vi "GetWindowParent.vi"(8 "No Error":errorcluster, 11 "Window [SDL_Window *]":i64) -> (0 "error out":errorcluster, 3 "Parent Window [SDL_Window *]":i64)   [LabVIEW 2024, in "SDL3.lvlib" / "Video.lvlib"]
doc: "<B>Summary</B>\nGet parent of a window."
uses:
  Video.lvlib
  Lib/SDL3-32.dll
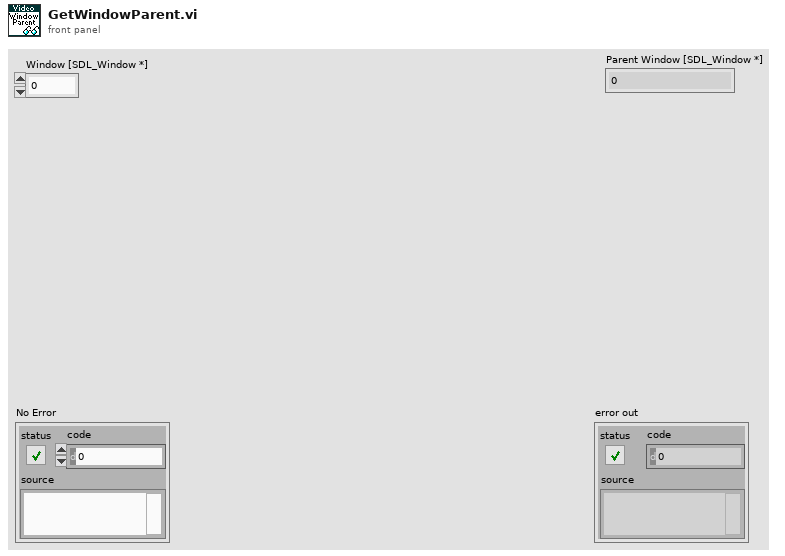
[diagram p1: front panel]
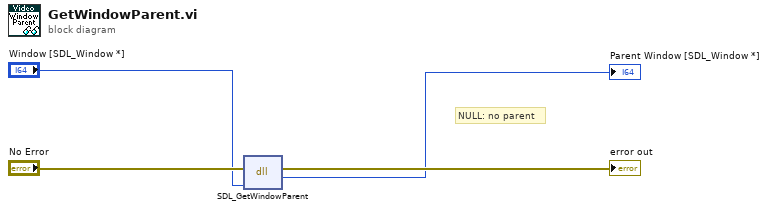
[diagram p0: block diagram]
diagram:
  # "NULL: no parent"
  n1 = dll-call lib="C:/Users/Thomas/Documents/Projects/LV-SDL3/Lib/SDL3-*.*" fn="SDL_GetWindowParent"(error in="No Error", "window"="Window [SDL_Window *]") -> (error out=→"error out":errorcluster, "return type"=→"Parent Window [SDL_Window *]":i64)  [unwired: 3 in, 1 out]
